vi "Send Set Sparse Marker Indexes [SM].vi"(7 "Message Priority (Normal)":T1=enum."Normal", 8 "error in (no error)":errorcluster, 9 "Indexes Array":i64[](array[numeric]) caption="indexes array", 10 "Marker Name (\"\")":string caption="marker name (\"\")", 11 "Message Enqueuer":refnum<class "Message Enqueuer.lvclass">) -> (0 "error out":errorcluster, 3 "Message Enqueuer out":refnum<class "Message Enqueuer.lvclass">)   [LabVIEW 2016, in "CS++Fgen.lvlib" / "Set Sparse Marker Indexes [SM] Msg.lvclass"]
doc: "Sends the <B>CS++Fgen.lvlib:Set Sparse Marker Indexes [SM] Msg.lvclass</B> message.\n\n<B>CS++Fgen.lvlib:CS++Fgen.lvclass:Set Sparse Marker Indexes [SM].vi</B> Description:\n\nThe VI sets the indexes associated with the sparse marker. These indexes may be coerced by the driver. Use the IviFgen Get Sparse Marker Indexes [SM] VI to find the coerced values.\n\nNote:\n\n(1) This VI is part of the IviFgenSparseMarker [SM] extension group."
uses:
  Set Sparse Marker Indexes [SM] Msg.lvclass
  <vilib>/ActorFramework/Message Enqueuer/Message Enqueuer.lvclass
  <vilib>/ActorFramework/Message Enqueuer/Message Priority.ctl
  C:/Program Files (x86)/National Instruments/LabVIEW 2016/vi.lib/ActorFramework/Message/Message.lvclass
  Set Sparse Marker Indexes [SM] Msg.lvclass/Set Sparse Marker Indexes [SM] Msg.ctl
  <vilib>/ActorFramework/Message Enqueuer/Message Enqueuer.lvclass/Message Enqueuer.ctl
  <vilib>/ActorFramework/Message Priority Queue/Priority Enqueue.vi
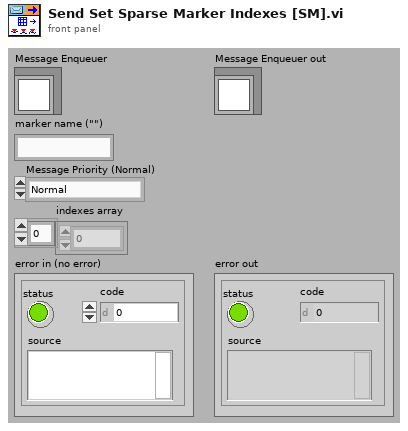
[diagram p1: front panel]
types:
  T1 = typedef "Actor Framework.lvlib/Message Enqueuer.lvclass/Message Priority.ctl" = enum16{"Low", "Normal", "High"}
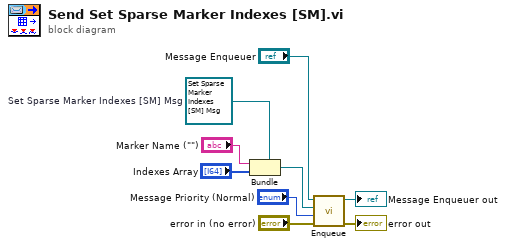
[diagram p0: block diagram]
diagram:
  w3 = refnum<class "Set Sparse Marker Indexes [SM] Msg.lvclass"> refnum  # Set Sparse Marker Indexes [SM] Msg
  n1 = Bundle(cluster=w3, "Marker Name (\"\")", "Indexes Array") -> (w6:refnum<class "Set Sparse Marker Indexes [SM] Msg.lvclass">)
  n2 = call <vilib>:"Enqueue.vi"("error in (no error)"="error in (no error)", "Message Priority (Normal)"="Message Priority (Normal)", "Message"=w6, "Message Enqueuer in"="Message Enqueuer") -> ("error out"=→"error out":errorcluster, "Message Enqueuer out"=→"Message Enqueuer out":refnum<class "Message Enqueuer.lvclass">)  [unwired: 6 in]
